vi "FTW-STR-Random-Hex.vi"(3 "String Length":i32=32) -> (0 "Random Hex String":string)   [LabVIEW 2015]
panel:
  # "Inputs"
  # "Outputs"
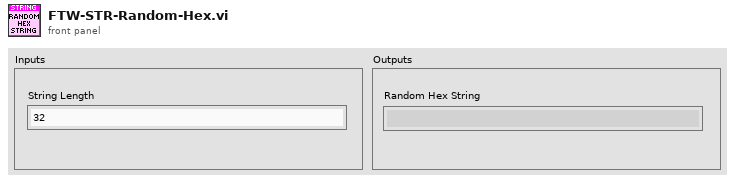
[diagram p1: front panel]
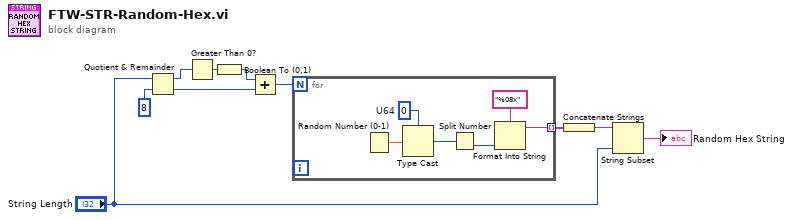
[diagram p0: block diagram]
diagram:
  n1 = Quotient & Remainder(x="String Length", y=8) -> (x-y*floor(x/y)=w5:i32, floor(x/y)=w2:i32)
  n2 = Greater Than 0?(x=w5) -> (x > 0?=w4:bool)
  n3 = Boolean To (0,1)(Boolean=w4) -> (0, 1=w3:i16)
  n4 = Add(x=w3, y=w2) -> (x+y=w1:i32)
  n5 = for {
    N: w1 -> [_]
    tunnel: [w11] -> w7 mode=indexing
    w15 = u64 0  # U64
    n6 = Random Number (0-1)() -> (number: 0 to 1=w12:dbl)
    n7 = Type Cast(type=w15, x=w12) -> (*(type *) &x=w14:u64)
    n8 = Split Number(x=w14) -> (lo(x)=w13:u32)  [unwired: 1 out]
    n9 = Format Into String(format string="%08x", w13) -> (resulting string=w11:string)  [unwired: 2 in, 1 out]
  }
  n10 = Concatenate Strings(w7) -> (w6:string)
  n11 = String Subset(string=w6, length (rest)="String Length") -> (substring=→"Random Hex String":string)  [unwired: 1 in]
